vi "Find Key Values.vi"(12 "error in":errorcluster) -> ()   [LabVIEW 2015]
uses:
  <vilib>/Utility/config.llb/Config Data RefNum.ctl
  <vilib>/Rock Robotics/Network Tables/NT Read String.vi
  <vilib>/Rock Robotics/Network Tables/NT Write Number.vi
  <vilib>/Rock Robotics/Network Tables/NT Write String.vi
  <vilib>/regexp/Match Regular Expression.xnode
  <vilib>/Utility/config.llb/NI_LVConfig.lvlib
panel:
  out "refnum":T1
  out "String":string
  out "Preferences":string[][](array[string])
  in  "stop":bool
  in  "Possible Choices":i32(ring)=1 items=["Hue1", "Hue2"]
  out "Value":string="NA"
  out "Key":string="NA"
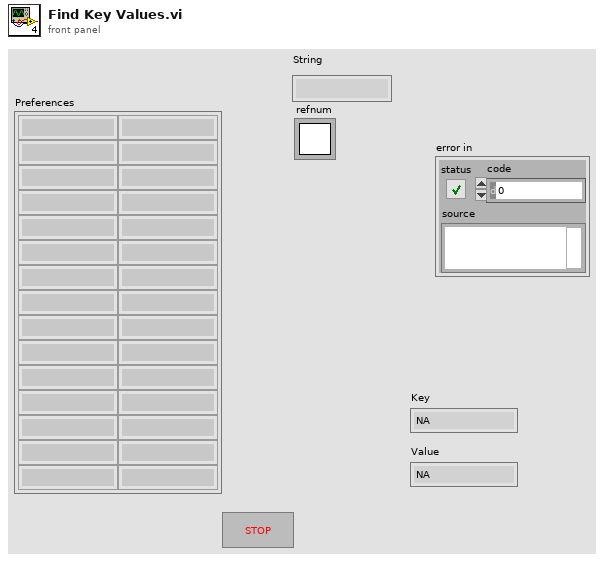
[diagram p1: front panel]
types:
  T1 = typedef "NI_LVConfig.lvlib/Config Data RefNum.ctl" = refnum<k1>
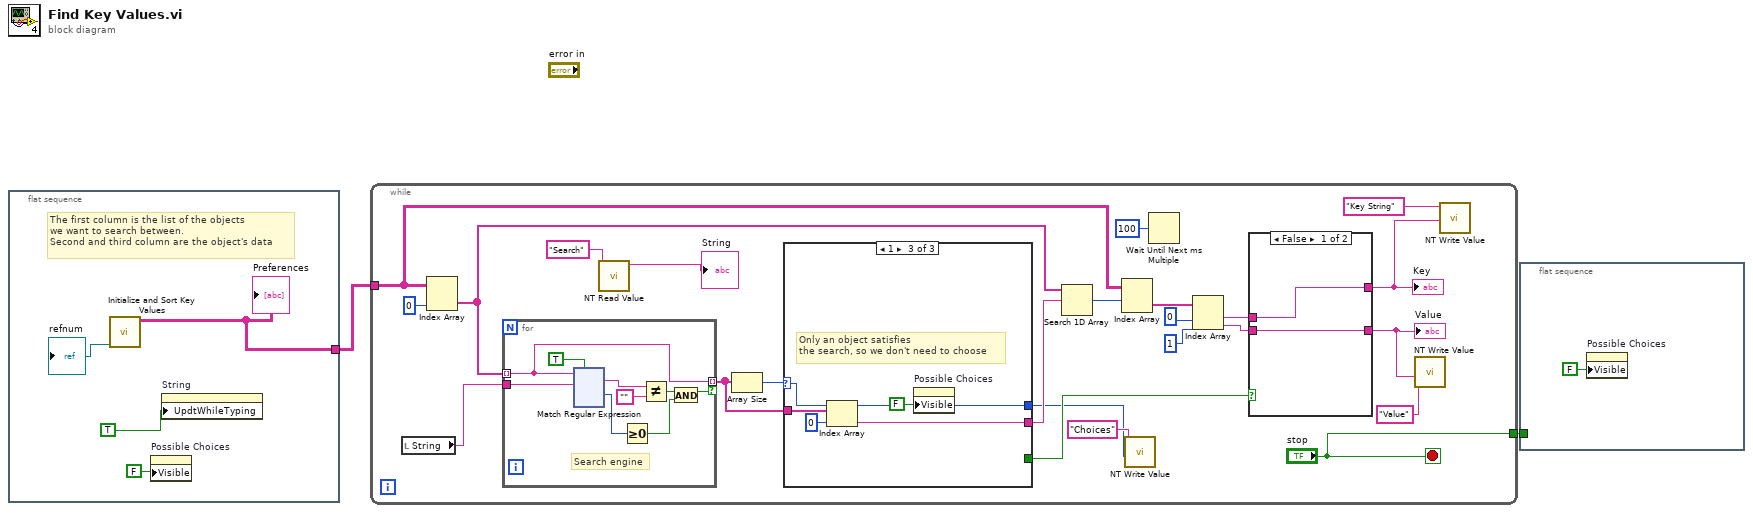
[diagram p0: block diagram]
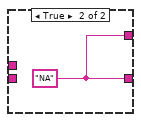
[diagram p2: hidden frame]
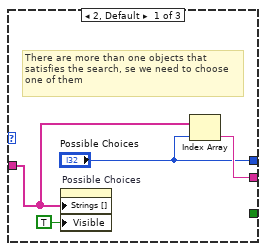
[diagram p3: hidden frame]
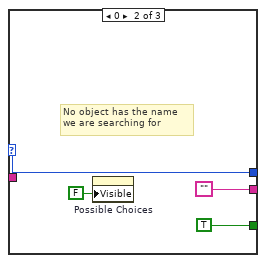
[diagram p4: hidden frame]
diagram:
  n1 = flat-sequence {
    tunnel: [w4] -> w2
    frame #0 {
      # "The first column is the list of the objects \nwe want to search between.\nSecond and third column are the object's data"
      n2 = call "Initialize and Sort Key Values.vi"() -> ("refnum"=→"refnum":T1, "Preferences"=w4:string[][])  [unwired: 10 in]
      "Preferences" <- w4
      n3 = property on="Possible Choices" class="Ring (strict)"("Visible"=FALSE) -> ()  [unwired: 2 in, 2 out]
      n4 = property on="String" class="Str"("UpdtWhileTyping"=TRUE ("Update While Typing?")) -> ()  [unwired: 2 in, 2 out]
    }
  }
  n5 = while {
    tunnel: w2 -> [w28]
    tunnel: ["stop"] -> w1
    stop <- "stop" stop-if-true
    n6 = local read "String"() -> (w15:string)
    n7 = Index Array(array=w28, index (col)=0 ("disabled index (col)")) -> (element=w25:string[])  [unwired: 1 in]
    n8 = for {
      tunnel: w15 -> [w55]
      tunnel: w25 -> [w51] mode=indexing
      tunnel: [w51] -> w26 mode=indexing if=w49
      # "Search engine"
      n9 = xnode "Match Regular Expression"("input string"=w51, "regular expression"=w55, "ignore case? (F)"=TRUE) -> ("whole match"=w53:string, "offset past match"=w50:i32)  [unwired: 3 in, 3 out]
      n10 = Greater Or Equal To 0?(x=w50) -> (x >= 0?=w48:bool)
      n11 = Not Equal?(x=w53, y="") -> (x != y?=w52:bool)
      n12 = And(x=w52, y=w48) -> (x .and. y?=w49:bool)
    }
    n13 = call-poly <vilib>:"NT Read Value.vi"("Name"="Search") -> ("String"=→"String":string)  [unwired: 9 in, 1 out]
    n14 = Array Size(array=w26) -> (size(s)=w27:i32)
    n15 = case shown="1" w27 {
      selector: w27 -> [_ w38 w42]
      tunnel: w26 -> [w37 _ w46]
      tunnel: [w36 "" w44] -> w24
      tunnel: [_ TRUE ("Visible") _] -> w18
      tunnel: ["Possible Choices" w38 w42] -> w13
      frame 2, Default {
        # "There are more than one objects that\nsatisfies the search, se we need to choose\none of them"
        n16 = property on="Possible Choices" class="Ring (strict)"("Strings []"=w37, "Visible"=TRUE) -> ()  [unwired: 2 in, 2 out]
        n17 = Index Array(array=w37, index="Possible Choices") -> (element=w36:string)
      }
      frame 0 {
        # "No object has the name \nwe are searching for"
        n18 = property on="Possible Choices" class="Ring (strict)"("Visible"=FALSE) -> ()  [unwired: 2 in, 2 out]
      }
      frame 1 {
        # "Only an object satisfies\nthe search, so we don't need to choose"
        n19 = Index Array(array=w46, index=0) -> (element=w44:string)
        n20 = property on="Possible Choices" class="Ring (strict)"("Visible"=FALSE) -> ()  [unwired: 2 in, 2 out]
      }
    }
    n21 = Search 1D Array(1D array=w25, element=w24) -> (index of element=w23:i32)  [unwired: 1 in]
    n22 = Index Array(array=w28, index (row)=w23) -> (element=w21:string[])  [unwired: 1 in]
    n23 = call-poly <vilib>:"NT Write Value.vi"("Numeric"=w13, "Name"="Choices") -> ()  [unwired: 9 in, 1 out]
    n24 = Wait Until Next ms Multiple(millisecond multiple=u32 100) -> ()  [unwired: 1 out]
    n25 = Index Array(array=w21, index #1=0 ("index"), index #2=1 ("index")) -> (element #1=w17:string, element #2=w16:string)
    n26 = case shown="False" w18 {
      tunnel: [w32 w33] -> w10
      tunnel: w17 -> [w32 _]
      tunnel: [w31 w33] -> w12
      tunnel: w16 -> [w31 _]
      frame False {
      }
      frame True {
        w33 = "NA" ("String")
      }
    }
    "Value" <- w12
    "Key" <- w10
    n27 = call-poly <vilib>:"NT Write Value.vi"("String"=w12, "Name"="Value") -> ()  [unwired: 9 in, 1 out]
    n28 = call-poly <vilib>:"NT Write Value.vi"("String"=w10, "Name"="Key String") -> ()  [unwired: 9 in, 1 out]
  }
  n29 = flat-sequence {
    tunnel: w1 -> [_]
    frame #0 {
      n30 = property on="Possible Choices" class="Ring (strict)"("Visible"=FALSE) -> ()  [unwired: 2 in, 2 out]
    }
  }
